vi "TSCAN_SetSignalValue_CAN.vi"(6 "SigValue":dbl, 7 "CANObJ IN":T1, 8 "错误输入（无错误）":errorcluster, 9 "Signal":string, 10 "CAN Message":string, 11 "路径输入":path) -> (0 "错误输出":errorcluster, 1 "CANObJ":T1, 2 "return":i32, 3 "路径输出":path)   [LabVIEW 2014]
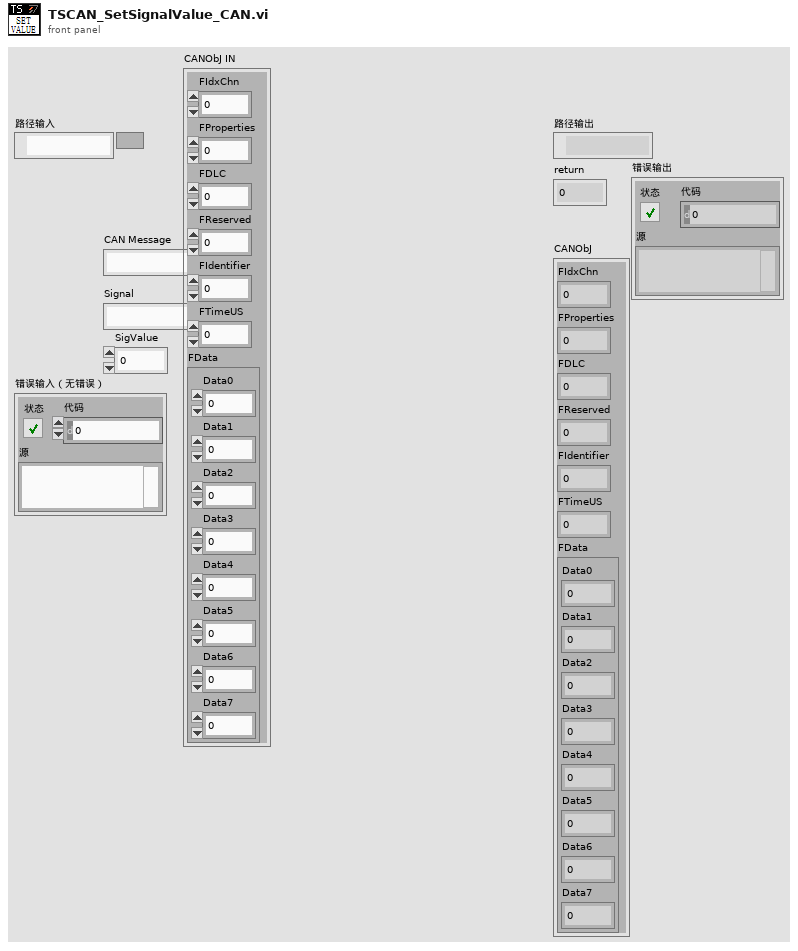
[diagram p1: front panel]
types:
  T1 = cluster{"FIdxChn":u8, "FProperties":u8, "FDLC":u8, "FReserved":u8, "FIdentifier":i32, "FTimeUS":u64, "FData":cluster{"Data0":u8, "Data1":u8, "Data2":u8, "Data3":u8, "Data4":u8, "Data5":u8, "Data6":u8, "Data7":u8}}
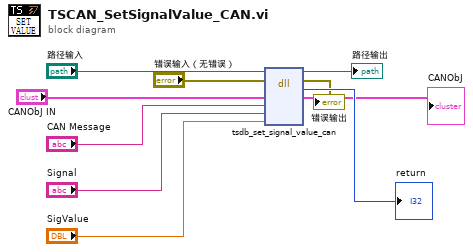
[diagram p0: block diagram]
diagram:
  n1 = dll-call lib="PTH27abs EDemo同星\nTSCAN_V1.0ConfigTSMaster.dll" fn="tsdb_set_signal_value_can"(path in="路径输入", error in="错误输入（无错误）", "CANObJ"="CANObJ IN", "Message"="CAN Message", "Signal"="Signal", "SigValue"="SigValue") -> (path out=→"路径输出":path, error out=→"错误输出":errorcluster, "tsdb_get_signal_value_can"=→"return":i32, "CANObJ"=→"CANObJ":T1)  [unwired: 4 in]
